vi "ATF-Pump-AO_Scale_Config.vi"(8 "error in (no error)":errorcluster, 10 "AO config":T1(array[cluster]), 11 "Refnum in":refnum<k21>) -> (0 "error out":errorcluster, 1 "Channel names":string[](array[string]), 2 "Default Value":dbl[](array[numeric]), 3 "Refnum out":refnum<k21>)   [LabVIEW 2022 SP3]
uses:
  <vilib>/DAQmx/create/channels.llb/DAQmx Create Channel (AO-Voltage-Basic).vi
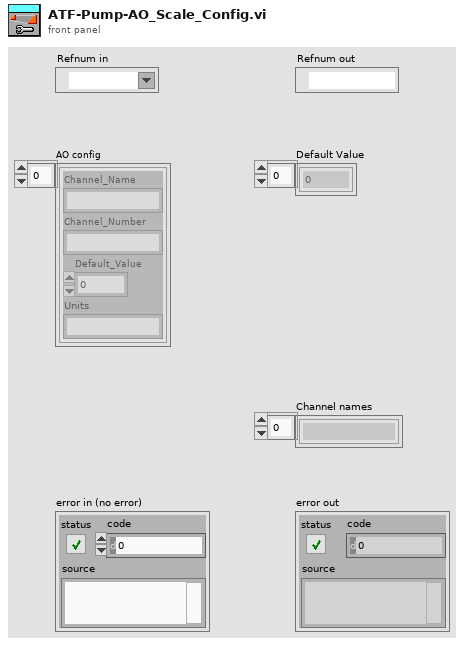
[diagram p1: front panel]
types:
  T1 = cluster{"Channel_Name":string, "Channel_Number":string, "Default_Value":dbl, "Units":string}[]
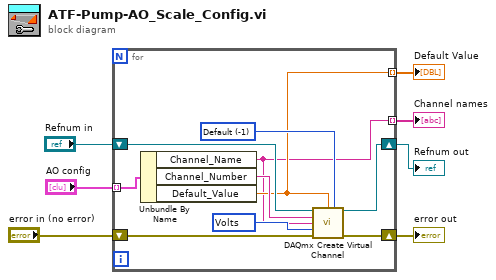
[diagram p0: block diagram]
diagram:
  n1 = for {
    shift-right: [w16] -> w4
    shift-left: "error in (no error)" -> [w11]
    tunnel: "AO config" -> [w14] mode=indexing
    shift-right: [w17] -> w5
    shift-left: "Refnum in" -> [w13]
    tunnel: [w9] -> w2 mode=indexing
    tunnel: [w8] -> w1 mode=indexing
    w10 = -1 items=["Default"=-1, "RSE"=10083, "Differential"=10106, "Pseudodifferential"=12529] ("output terminal configuration")
    w15 = 10348 items=["Volts"=10348, "From Custom Scale"=10065] ("units")
    n2 = Unbundle By Name(w14) -> ("Channel_Name"=w8:string, "Channel_Number"=w12:string, "Default_Value"=w9:dbl)
    n3 = call-poly <vilib>:"DAQmx Create Virtual Channel.vi"("task in"=w13, "minimum value"=w9, "output terminal configuration"=w10, "physical channels"=w12, "name to assign"=w8, "units"=w15, "error in"=w11) -> ("task out"=w17:refnum<k21>, "error out"=w16:errorcluster)  [unwired: 7 in]
  }
  "Refnum out" <- w5
  "error out" <- w4
  "Default Value" <- w2
  "Channel names" <- w1
